vi "CFTS-Read state.vi"(0 "State In":T1, 11 "error in (no error)":errorcluster) -> (4 "State Out":T1, 15 "error out":errorcluster)   [LabVIEW 2020]
uses:
  CFTS-Experiment State.ctl
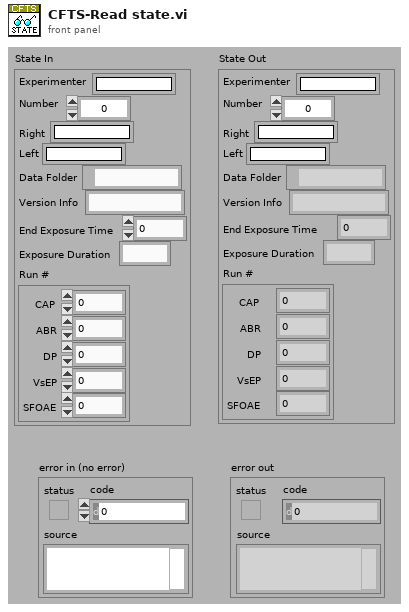
[diagram p1: front panel]
types:
  T1 = typedef "CFTS-Experiment State.ctl" = cluster{"Experimenter":string, "Number":u32, "Right":string, "Left":string, "Data Folder":path, "Version Info":string, "End Exposure Time":dbl, "Exposure Duration":string, "Run #":cluster{"CAP":i32, "ABR":i32, "DP":i32, "VsEP":i32, "SFOAE":i32}}
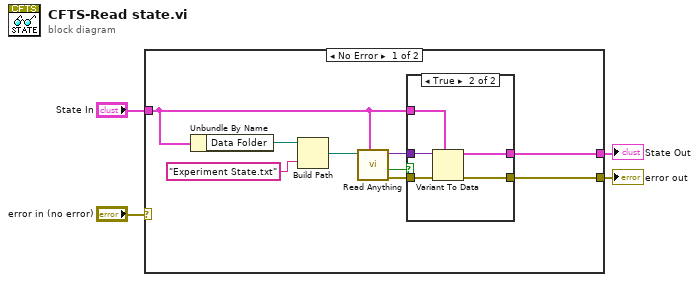
[diagram p0: block diagram]
diagram:
  n1 = case shown="No Error" "error in (no error)" {
    selector: "error in (no error)" -> [_ w21]
    tunnel: [w6 w21] -> w4
    tunnel: [w7 w22] -> w1
    tunnel: "State In" -> [w8 w22]
    frame No Error {
      n2 = Unbundle By Name(w8) -> ("Data Folder"=w13:path)
      n3 = Build Path(base path=w13, name or relative path="Experiment State.txt") -> (appended path=w11:path)
      n4 = call "Read Anything.vi"("Type of Anything"=w8, "Path (dialog)"=w11) -> ("Error Out"=w10:errorcluster, "Found?"=w9:bool, "Anything"=w5:variant)  [unwired: 7 in]
      n5 = case shown="True" w9 {
        tunnel: w10 -> [w14 w20]
        tunnel: w8 -> [w15 w19]
        tunnel: [w15 w18] -> w7
        tunnel: [w14 w17] -> w6
        tunnel: w5 -> [_ w16]
        frame False {
        }
        frame True {
          n6 = Variant To Data(error in=w20, type=w19, Variant=w16) -> (data=w18:T1, error out=w17:errorcluster)
        }
      }
    }
    frame Error {
    }
  }
  "error out" <- w4
  "State Out" <- w1
